vi "Unwind.vi"(8 "Error In":errorcluster, 11 "AutoData":T1) -> (0 "Error Out":errorcluster, 3 "AutoData out":T1)   [LabVIEW 2019, in "AutoMode.lvlib"]
uses:
  AutoMode.lvlib
  Cluster - AutoModeData.ctl
  MainController/Cluster - TestSettings.ctl
  MainController/Cluster - HardwareConfiguration.ctl
  MainController/Cluster - TestResults.ctl
  Cluster - AutoModeMessage.ctl
  Enum - AutoModeState.ctl
  MainController/Cluster - MainControllerMessage.ctl
  MainController/Enum - MainState.ctl
  Mark10 API/WriteSpeed.vi
  Mark10 API/WriteCWTravelLimit.vi
  Mark10 API/WriteMoveTestStandCW.vi
  Mark10 API/Mark 10 TSTM-DC.lvlib
  Timer/Timer.lvlib
  EventLogger/EventLogger.lvlib
  MainController/MainController.lvlib
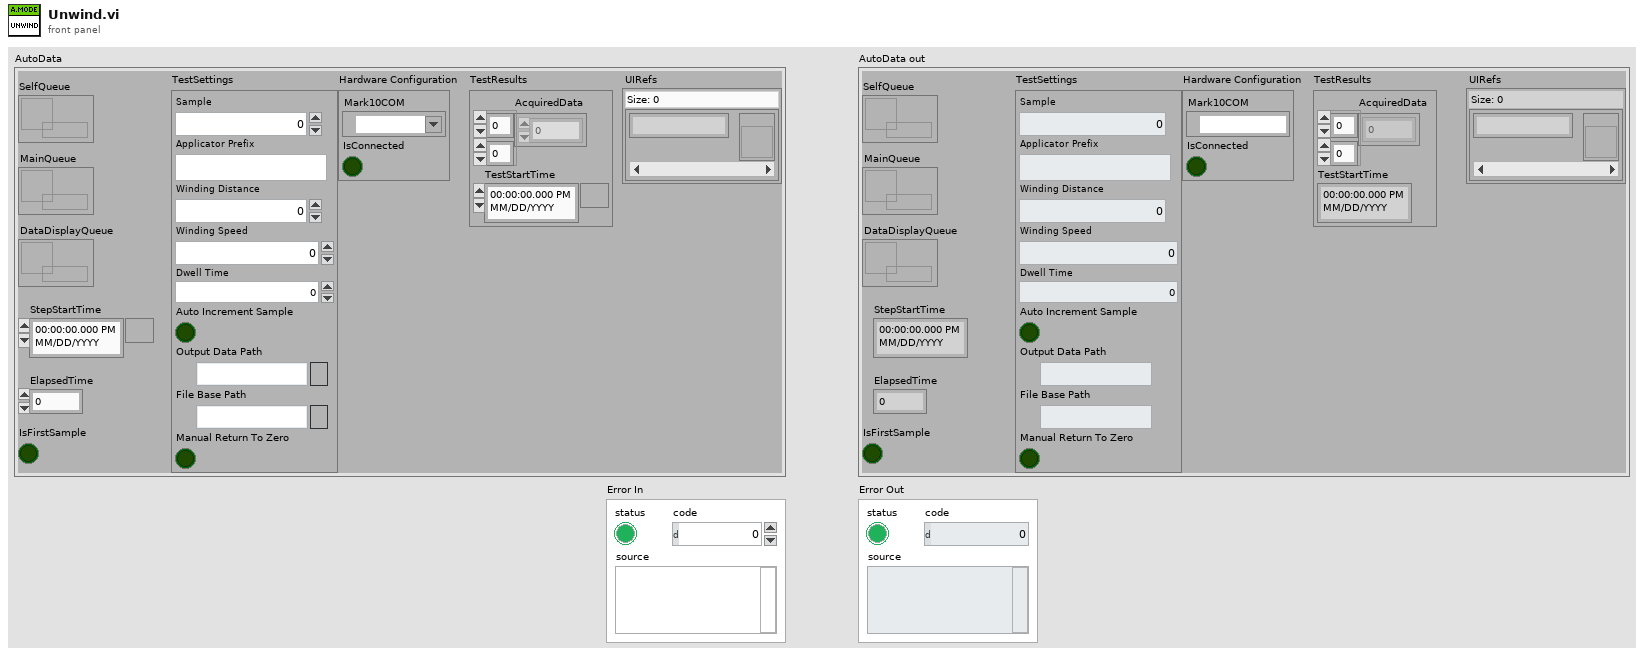
[diagram p1: front panel]
types:
  T1 = typedef "AutoMode.lvlib/Cluster - AutoModeData.ctl" = cluster{"DataDisplayQueue":refnum<queue>, "StepStartTime":timestamp, "TestSettings":T2, "Hardware Configuration":T3, "TestResults":T4, "ElapsedTime":dbl, "IsFirstSample":bool, "SelfQueue":refnum<queue>, "MainQueue":refnum<queue>, "UIRefs":map{string, refnum<vi>}}
  T2 = typedef "MainController.lvlib/Cluster - TestSettings.ctl" = cluster{"Sample":u32, "Applicator Prefix":string, "Winding Distance":dbl, "Winding Speed":dbl, "Dwell Time":dbl, "Auto Increment Sample":bool, "Output Data Path":path, "File Base Path":path, "Manual Return To Zero":bool}
  T3 = typedef "MainController.lvlib/Cluster - HardwareConfiguration.ctl" = cluster{"Mark10COM":refnum<visa-resource-name>, "IsConnected":bool}
  T4 = typedef "MainController.lvlib/Cluster - TestResults.ctl" = cluster{"AcquiredData":dbl[][], "TestStartTime":timestamp}
  T5 = typedef "AutoMode.lvlib/Enum - AutoModeState.ctl" = enum16{"Initialize", "Idle", "UpdateConfig", "UpdateHWConfig", "BroadcastSettings", "Start", "CheckValidReportPath", "Winding", "WaitForWinding", "Unwind", "WaitForUnwind", "Stop", "Abort", "WriteDataToFile", "EventTriggered", "GenerateFilePath", "ZeroPosition", "GotoZero", "Error", "Exit"}
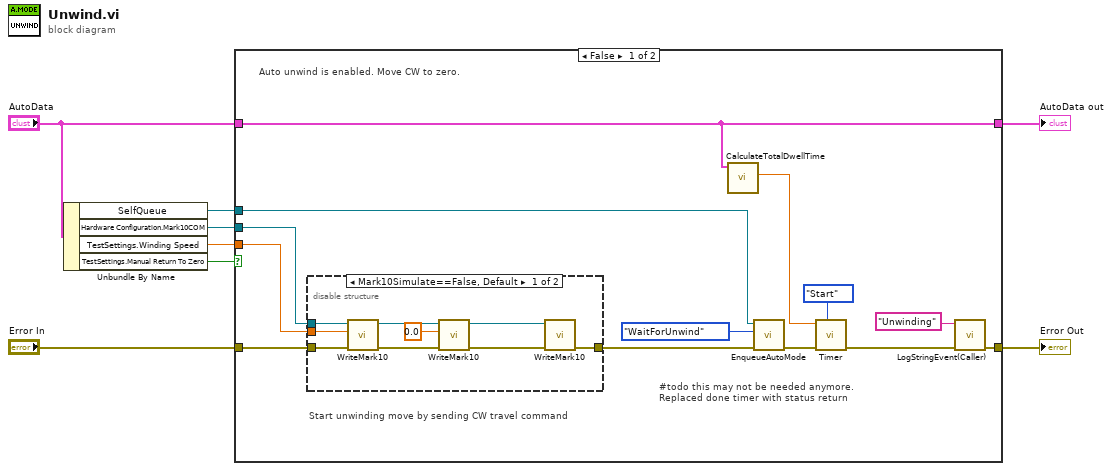
[diagram p0: block diagram]
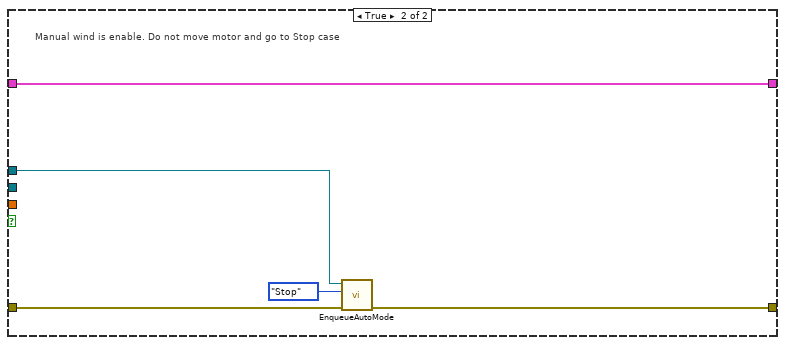
[diagram p3: hidden frame]
diagram:
  n1 = Unbundle By Name("AutoData") -> ("SelfQueue"=w4:refnum<queue>, "Hardware Configuration.Mark10COM"=w8:refnum<visa-resource-name>, "TestSettings.Winding Speed"=w3:dbl, "TestSettings.Manual Return To Zero"=w2:bool)
  n2 = case shown="False" w2 {
    tunnel: w8 -> [w19 _]
    tunnel: "Error In" -> [w15 w35]
    tunnel: [w10 w34] -> w6
    tunnel: "AutoData" -> [w11 w36]
    tunnel: w4 -> [w13 w33]
    tunnel: w3 -> [w12 _]
    tunnel: [w11 w36] -> w1
    frame False {
      # "Auto unwind is enabled. Move CW to zero."
      # "#todo this may not be needed anymore.\nReplaced done timer with status return"
      # "Start unwinding move by sending CW travel command"
      n3 = disable-structure shown="Mark10Simulate==False, Default" {
        disable-tunnel: [w30 w31] -> w21
        disable-tunnel: w15 -> [w29 w31]
        disable-tunnel: w19 -> [w24 _]
        disable-tunnel: w12 -> [w22 _]
        frame condition #0 (active) {
          n4 = call-poly "WriteMark10.vi"("error in"=w29, "Speed"=w22, "VISA resource name"=w24) -> ("error out"=w25:errorcluster, "VISA resource name out"=w23:refnum<visa-resource-name>)  [unwired: 7 in]
          n5 = call-poly "WriteMark10.vi"("error in"=w25, "CWTravelLimit"=0.0, "VISA resource name"=w23) -> ("error out"=w27:errorcluster, "VISA resource name out"=w28:refnum<visa-resource-name>)  [unwired: 7 in]
          n6 = call-poly "WriteMark10.vi"("error in"=w27, "VISA resource name"=w28) -> ("error out"=w30:errorcluster)  [unwired: 8 in, 1 out]
        }
        frame condition #1 {
        }
      }
      n7 = call "CalculateTotalDwellTime.vi"("AutoData"=w11) -> ("DwellTime"=w16:dbl)  [unwired: 10 in]
      n8 = call "EnqueueAutoMode.vi"("error in (no error)"=w21, "AutoState"=Enum_-_AutoModeState."WaitForUnwind" ("CycleTestState"), "Queue in"=w13) -> ("error out"=w18:errorcluster)  [unwired: 7 in, 1 out]
      n9 = call "Timer.vi"("TimerState"=enum16{"Reset", "Start", "GetTime", "Stop"}."Start", "Error In"=w18, "TargetTime(ms)"=w16) -> ("Error Out"=w14:errorcluster)  [unwired: 7 in, 1 out]
      n10 = call "LogStringEvent(Caller).vi"("Error In"=w14, "Field"="Unwinding") -> ("Error Out"=w10:errorcluster)  [unwired: 9 in]
    }
    frame True {
      # "Manual wind is enable. Do not move motor and go to Stop case"
      n11 = call "EnqueueAutoMode.vi"("error in (no error)"=w35, "AutoState"=Enum_-_AutoModeState."Stop", "Queue in"=w33) -> ("error out"=w34:errorcluster)  [unwired: 7 in, 1 out]
    }
  }
  "Error Out" <- w6
  "AutoData out" <- w1
